vi "认识公式节点.vi"() -> ()   [LabVIEW 2018]
panel:
  in  "停止":bool
  out "sub":dbl
  out "add":dbl
  in  "输入变量b":dbl
  in  "输入变量i":dbl
  out "字符串":string
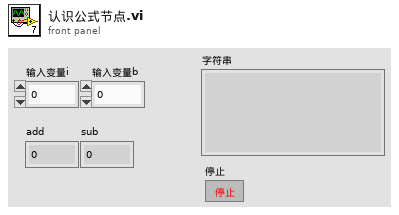
[diagram p1: front panel]
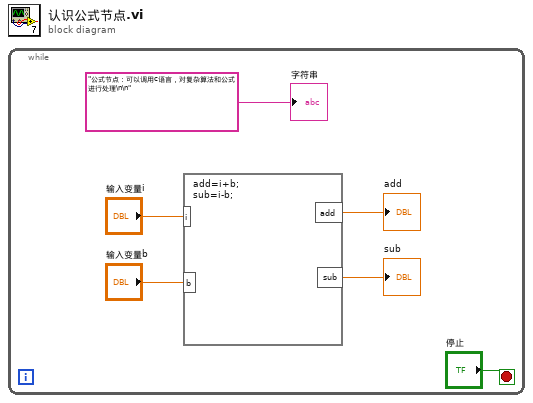
[diagram p0: block diagram]
diagram:
  n1 = while {
    stop <- "停止" stop-if-true
    n2 = formula code="add=i+b;\nsub=i-b;"("i"="输入变量i", "b"="输入变量b") -> ("add"=→"add":dbl, "sub"=→"sub":dbl)
    "字符串" <- "公式节点：可以调用c语言，对复杂算法和公式进行处理\n\n"
  }
